vi "DDS_use_sub_vi.vi"() -> ()   [LabVIEW 2012]
panel:
  in  "Channel":u16(ring) items=["DDS_0", "DDS_1"]
  in  "Amplitude (dBm)":dbl=-5.0 min=-63.0 max=-5.0 step=0.01 format="%_4g"
  in  "Frequency (MHz)":dbl=80.0 min=10.0 max=150.0 step=1e-09 format="%.9f"
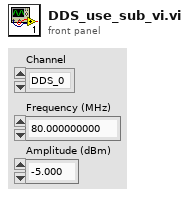
[diagram p1: front panel]
types:
  T1 = cluster{"address":string, "port":u16, "password":string}
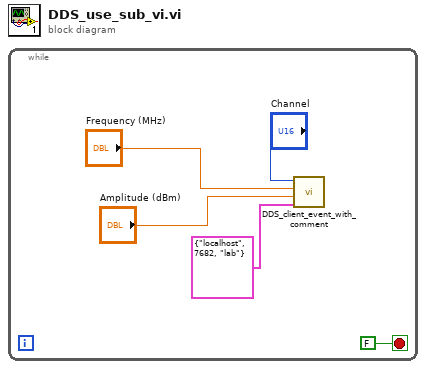
[diagram p0: block diagram]
diagram:
  n1 = while {
    stop <- FALSE stop-if-true
    n2 = call "DDS_client_event_with_comment.vi"("manager"=T1 {"address"="localhost", "port"=7682, "password"="lab"}, "Amplitude (dBm)"="Amplitude (dBm)", "Frequency (MHz)"="Frequency (MHz)", "Channel"="Channel") -> ()  [unwired: 8 in]
  }
